vi "2x3CIM Open.vi"(0 "RightMotor1":T1, 1 "RightMotor2":T1, 2 "RightMotor3":T1, 3 "RightMotorsInverted":bool, 11 "LeftMotor1":T1, 12 "LeftMotor2":T1, 13 "LeftMotor3":T1, 14 "LeftMotorsInverted":bool, 15 "error in":errorcluster) -> (4 "error out":errorcluster)   [LabVIEW 2015]
doc: "Configures Talon SRXes without CAN for use with two VexPro WCP DS 3-CIM Assemblies. The third CIM on each assembly is inverted due to gearbox design, and the others are interchangeable."
uses:
  <vilib>/Rock Robotics/SystemInterfaces/DIO/FPGA_DIOPWMChannel.ctl
  <vilib>/Rock Robotics/WPI/MotorControl/WPI_MotorControlOpen TalonSRX.vi
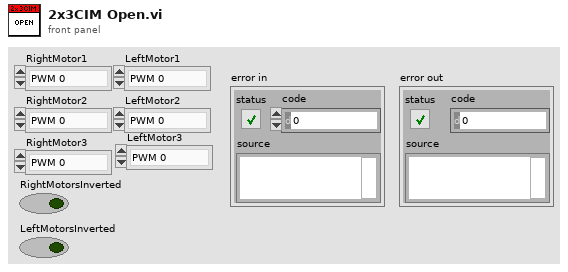
[diagram p1: front panel]
types:
  T1 = typedef "FPGA_DIOPWMChannel.ctl" = enum8{"PWM 0", "PWM 1", "PWM 2", "PWM 3", "PWM 4", "PWM 5", "PWM 6", "PWM 7", "PWM 8", "PWM 9", "PWM MXP 0", "PWM MXP 1", "PWM MXP 2", "PWM MXP 3", "PWM MXP 4", "PWM MXP 5", "PWM MXP 6", "PWM MXP 7", "PWM MXP 8", "PWM MXP 9", "Invalid"}
  T2 = typedef "WPI_MotorControlDeviceRef.ctl" = cluster{"DeviceStatus":errorcluster, "Type":T3, "PWM":cluster{"PWM Channel":T1, "DeadBand":T4}, "CAN":cluster{"Device Number":u8, "Control Mode":T5, "Semaphore":T6, "Max Vout":dbl, "TalonSRX Control Mode":T7}, "Invert":bool}
  T3 = typedef "WPI_MotorControlType.ctl" = enum16{"PWM", "CAN", "CANTalonSRX"}
  T4 = typedef "WPI_PWMDeadband.ctl" = cluster{"Name":string, "maxPositivePwm":i32, "minPositivePwm":i32, "centerPwm":i32, "maxNegativePwm":i32, "minNegativePwm":i32, "angularRange":u16}
  T5 = typedef "WPI_CANJaguar_ControlMode.ctl" = enum8{"Percent VBus", "Current", "Speed", "Position", "Voltage"}
  T6 = typedef "Semaphore RefNum" = refnum<k1>
  T7 = typedef "WPI_CANTalonSRX_APIControlMode.ctl" = enum8{"Percent VBus", "Speed", "Position", "Slave", "Unchanged / Invalid", "Voltage Compensation", "Current", "Motion Profile"}
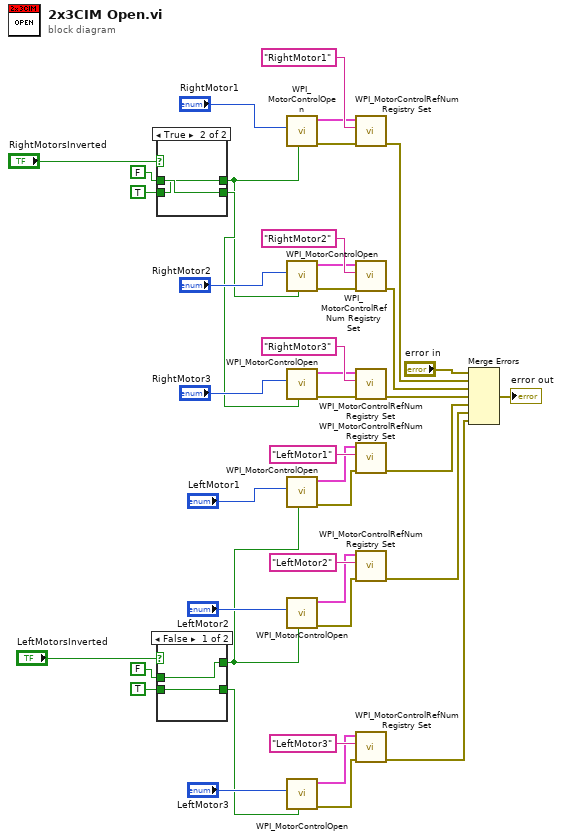
[diagram p0: block diagram]
diagram:
  n1 = case shown="True" "RightMotorsInverted" {
    tunnel: [w44 w45] -> w6
    tunnel: FALSE -> [w44 w46]
    tunnel: [w43 w46] -> w9
    tunnel: TRUE -> [w43 w45]
    frame False {
    }
    frame True {
    }
  }
  n2 = case shown="False" "LeftMotorsInverted" {
    tunnel: [w47 w50] -> w8
    tunnel: FALSE -> [w48 w50]
    tunnel: [w48 w49] -> w7
    tunnel: TRUE -> [w47 w49]
    frame False {
    }
    frame True {
    }
  }
  n3 = call-poly <vilib>:"WPI_MotorControlOpen.vi"("Invert"=w6, "PWM Channel"="RightMotor1") -> ("error out"=w37:errorcluster, "MotorControlDeviceRef"=w30:T2)  [unwired: 8 in]
  n4 = call-poly <vilib>:"WPI_MotorControlOpen.vi"("Invert"=w6, "PWM Channel"="RightMotor2") -> ("error out"=w38:errorcluster, "MotorControlDeviceRef"=w29:T2)  [unwired: 8 in]
  n5 = call-poly <vilib>:"WPI_MotorControlOpen.vi"("Invert"=w9, "PWM Channel"="RightMotor3") -> ("error out"=w39:errorcluster, "MotorControlDeviceRef"=w28:T2)  [unwired: 8 in]
  n6 = call-poly <vilib>:"WPI_MotorControlOpen.vi"("Invert"=w7, "PWM Channel"="LeftMotor1") -> ("error out"=w40:errorcluster, "MotorControlDeviceRef"=w27:T2)  [unwired: 8 in]
  n7 = call-poly <vilib>:"WPI_MotorControlOpen.vi"("Invert"=w7, "PWM Channel"="LeftMotor2") -> ("error out"=w41:errorcluster, "MotorControlDeviceRef"=w26:T2)  [unwired: 8 in]
  n8 = call-poly <vilib>:"WPI_MotorControlOpen.vi"("Invert"=w8, "PWM Channel"="LeftMotor3") -> ("error out"=w42:errorcluster, "MotorControlDeviceRef"=w25:T2)  [unwired: 8 in]
  n9 = call <vilib>:"WPI_MotorControlRefNum Registry Set.vi"("error in (no error)"=w37, "refnum name"="RightMotor1", "MotorControlDevRef"=w30) -> ("error out"=w24:errorcluster)  [unwired: 7 in, 1 out]
  n10 = call <vilib>:"WPI_MotorControlRefNum Registry Set.vi"("error in (no error)"=w38, "refnum name"="RightMotor2", "MotorControlDevRef"=w29) -> ("error out"=w23:errorcluster)  [unwired: 7 in, 1 out]
  n11 = call <vilib>:"WPI_MotorControlRefNum Registry Set.vi"("error in (no error)"=w39, "refnum name"="RightMotor3", "MotorControlDevRef"=w28) -> ("error out"=w22:errorcluster)  [unwired: 7 in, 1 out]
  n12 = call <vilib>:"WPI_MotorControlRefNum Registry Set.vi"("error in (no error)"=w40, "refnum name"="LeftMotor1", "MotorControlDevRef"=w27) -> ("error out"=w21:errorcluster)  [unwired: 7 in, 1 out]
  n13 = call <vilib>:"WPI_MotorControlRefNum Registry Set.vi"("error in (no error)"=w41, "refnum name"="LeftMotor2", "MotorControlDevRef"=w26) -> ("error out"=w19:errorcluster)  [unwired: 7 in, 1 out]
  n14 = call <vilib>:"WPI_MotorControlRefNum Registry Set.vi"("error in (no error)"=w42, "refnum name"="LeftMotor3", "MotorControlDevRef"=w25) -> ("error out"=w20:errorcluster)  [unwired: 7 in, 1 out]
  n15 = Merge Errors("error in", w24, w23, w22, w21, w19, w20) -> (→"error out":errorcluster)
